vi "Destroy.vi"(8 "error in (no error)":errorcluster, 11 "ListImp in":refnum<class "ListImp.lvclass">) -> (0 "error out":errorcluster)   [LabVIEW 2013, in "LapDog.Collections.v_.Lists.lvlib" / "ListImp.lvclass"]
uses:
  ListImp.lvclass
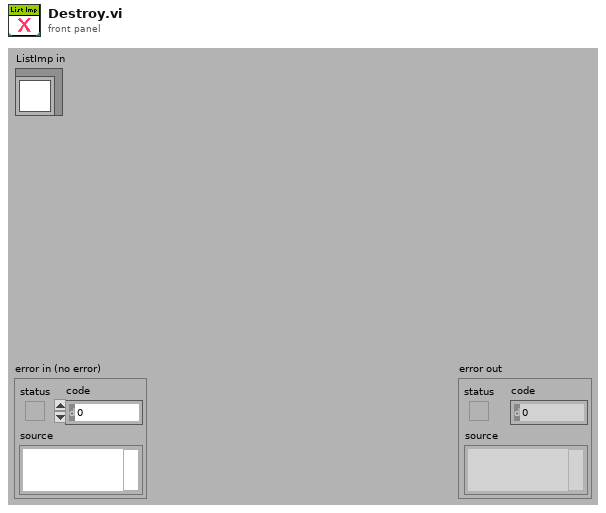
[diagram p1: front panel]
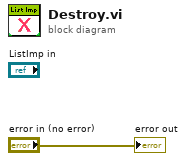
[diagram p0: block diagram]
diagram:
  "error out" <- "error in (no error)"
